vi "Is in range.vi"(8 "error in (no error)":errorcluster, 9 "Upper end":refnum<class "Mag Lab Result.lvclass">, 10 "Lower end":refnum<class "Mag Lab Result.lvclass">, 11 "Mag Lab Result in":refnum<class "Mag Lab Result.lvclass">) -> (0 "error out":errorcluster, 3 "Mag Lab Result out":refnum<class "Mag Lab Result.lvclass">, 4 "Is in range?":bool)   [LabVIEW 2015, in "Mag Lab Result.lvclass"]
uses:
  Mag Lab Result.lvclass
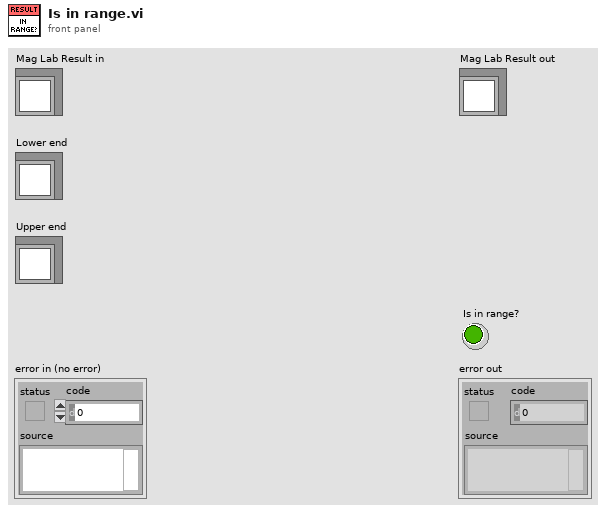
[diagram p1: front panel]
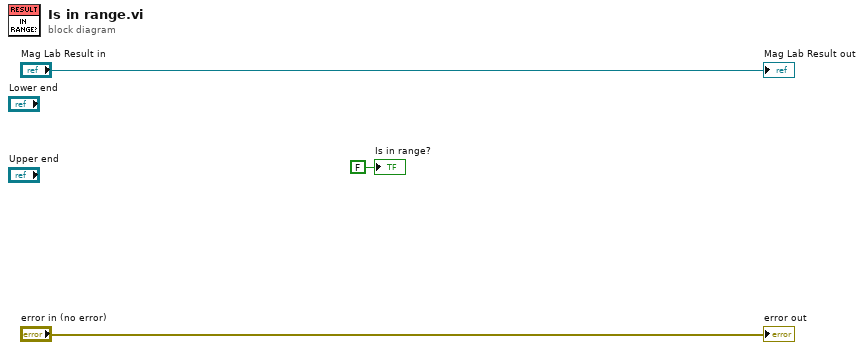
[diagram p0: block diagram]
diagram:
  "error out" <- "error in (no error)"
  "Mag Lab Result out" <- "Mag Lab Result in"
  "Is in range?" <- FALSE ("Is in range?")
